vi "Convert ExcelValues To Class.vi"(8 "error in (no error)":errorcluster, 10 "Excel Value(\"\")":string[][](array[string]), 11 "MemberTable in":refnum<class "TimeTable.lvclass">) -> (0 "error out":errorcluster, 3 "MemberTable out":refnum<class "TimeTable.lvclass">)   [LabVIEW 2015, in "TimeTable.lvclass"]
uses:
  TimeTable.lvclass
  Type Definitions/Table_Cell.ctl
  TimeTable.lvclass/TimeTable.ctl
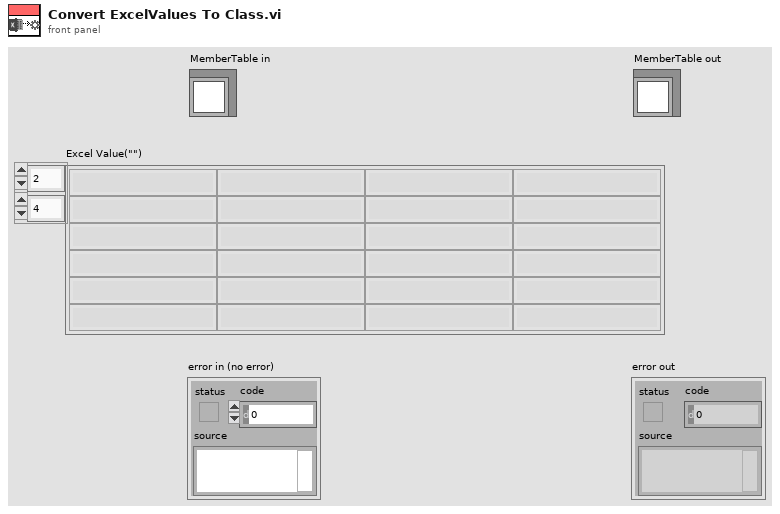
[diagram p1: front panel]
types:
  T1 = typedef "TimeTable.lvclass/Table_Cell.ctl" = cluster{"结束周":i32, "起始周":i32, "课程名称":string}
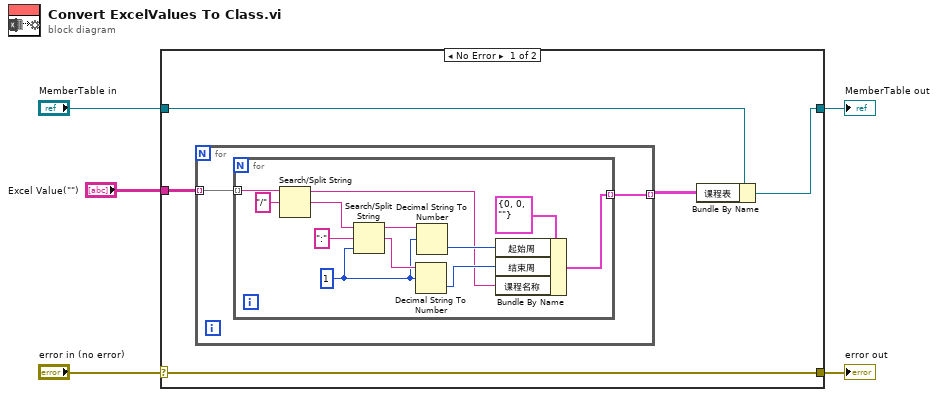
[diagram p0: block diagram]
diagram:
  n1 = case shown="No Error" "error in (no error)" {
    selector: "error in (no error)" -> [w10 w26]
    tunnel: [w10 w26] -> w4
    tunnel: [w6 w25] -> w2
    tunnel: "MemberTable in" -> [w8 w25]
    tunnel: "Excel Value(\"\")" -> [w9 _]
    frame No Error {
      n2 = for {
        tunnel: w9 -> [w12] mode=indexing
        tunnel: [w11] -> w7 mode=indexing
        n3 = for {
          tunnel: w12 -> [w24] mode=indexing
          tunnel: [w14] -> w11 mode=indexing
          w13 = 1 ("offset (0)")
          n4 = Search/Split String(string=w24, search string/char (-)="/") -> (substring before match=w15:string, match + rest of string=w22:string)  [unwired: 1 in, 1 out]
          n5 = Search/Split String(string=w22, search string/char (-)=":", offset (0)=w13) -> (substring before match=w18:string, match + rest of string=w17:string)  [unwired: 1 out]
          n6 = Decimal String To Number(string=w17, offset=w13) -> (number=w16:i32)  [unwired: 1 in, 1 out]
          n7 = Decimal String To Number(string=w18, offset=w13) -> (number=w19:i32)  [unwired: 1 in, 1 out]
          n8 = Bundle By Name(cluster=T1 {"结束周"=0, "起始周"=0, "课程名称"=""} ("课程格子"), "起始周"=w19, "结束周"=w16, "课程名称"=w15) -> (w14:T1)
        }
      }
      n9 = Bundle By Name(cluster=w8, "课程表"=w7) -> (w6:refnum<class "TimeTable.lvclass">)
    }
    frame Error {
    }
  }
  "error out" <- w4
  "MemberTable out" <- w2
